vi "Set Thru Paths.vi"(8 "error in (no error)":errorcluster {"code" format="%.0x"}, 9 "PortPath":i32[](array[numeric])=[0], 11 "instrument handle":refnum<k15>) -> (0 "error out":errorcluster {"code" format="%.0x"}, 3 "instrument handle out":refnum<k15>)   [LabVIEW 2014, in "Agilent NA.lvlib"]
doc: "Set the set of thru paths to be calibrated."
uses:
  Agilent NA.lvlib
  AgNA.dll
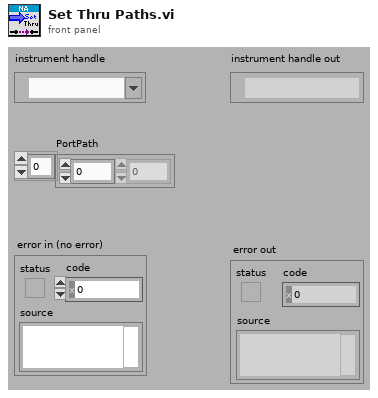
[diagram p1: front panel]
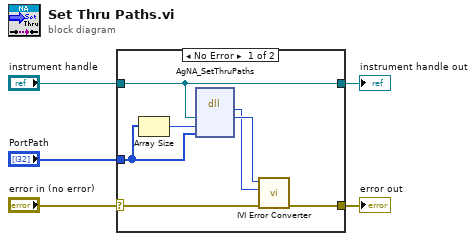
[diagram p0: block diagram]
diagram:
  n1 = case shown="No Error" "error in (no error)" {
    selector: "error in (no error)" -> [w10 w14]
    tunnel: [w9 w14] -> w5
    tunnel: "PortPath" -> [w7 _]
    tunnel: [w8 w13] -> w2
    tunnel: "instrument handle" -> [w8 w13]
    frame No Error {
      n2 = Array Size(array=w7) -> (size(s)=w6:i32)
      n3 = dll-call lib="AgNA**.dll" fn="AgNA_SetThruPaths"("Vi"=w8, "PortPathBufferSize"=w6, "PortPath"=w7) -> (w11:i32, "Vi"=w12:u32)  [unwired: 5 in, 2 out]
      n4 = call "IVI Error Converter.vi"("error in (no error)"=w10, "IVI error code (0)"=w11, "instrument handle"=w12) -> ("error out"=w9:errorcluster)  [unwired: 7 in, 1 out]
    }
    frame Error {
    }
  }
  "error out" <- w5
  "instrument handle out" <- w2
